vi "AVS_UseHighResADC.vi"(1 "a_Enable":u8, 2 "a_hDevice":i32) -> (0 "Output Value":i32)   [LabVIEW 2013, in "Avantes Spectrometer Functions.lvlib"]
uses:
  Avantes Spectrometer Functions.lvlib
  AS5216.dll
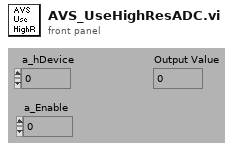
[diagram p1: front panel]
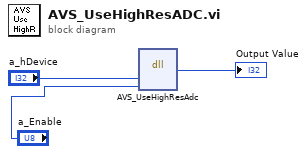
[diagram p0: block diagram]
diagram:
  n1 = dll-call lib="C:/Users/dhstuart/Dropbox/CLTC/avantesSpectrometer/Libraries/AS-5216-DLL/polling_mc/AS5216.dll" fn="AVS_UseHighResAdc"("a_hDevice"="a_hDevice", "a_Enable"="a_Enable") -> ("return type"=→"Output Value":i32)  [unwired: 5 in, 2 out]
